vi "Calculate_Angles_Locally_Optimum-1.vi"(4 "Statuses":i16[](array[numeric]), 5 "[IN] Index of subtrack":i32, 6 "[IN] Reverse Displ or Not":bool[](array[boolean]), 7 "[IN] Array with Angles \nBetween Displacement":dbl[](array[numeric]), 8 "[IN] Index of Cur\nrent Displacement":i32, 9 "[IN] Track with \nCurrent Point":dbl[](array[numeric]), 10 "[IN] Index of Previ\nous Displacement":i32, 11 "[IN] Track with \nPrevious Point":dbl[](array[numeric])) -> (1 "[OUT] Reverse displacement or not":bool[](array[boolean]), 2 "[OUT] Angles betwe\nen two displacements":dbl[](array[numeric]))   [LabVIEW 2013]
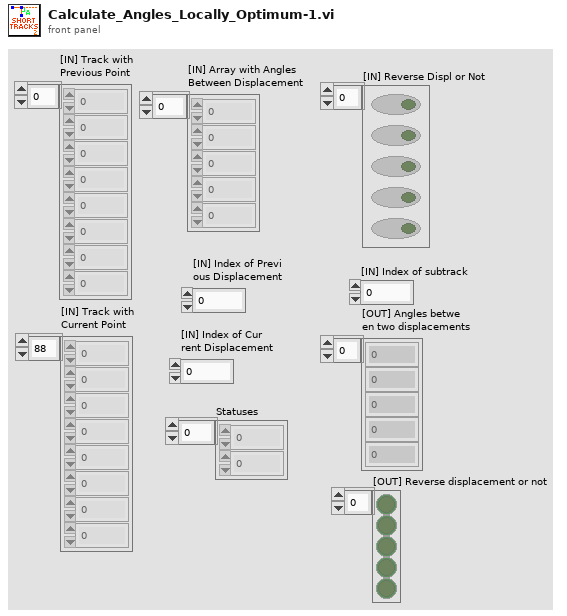
[diagram p1: front panel]
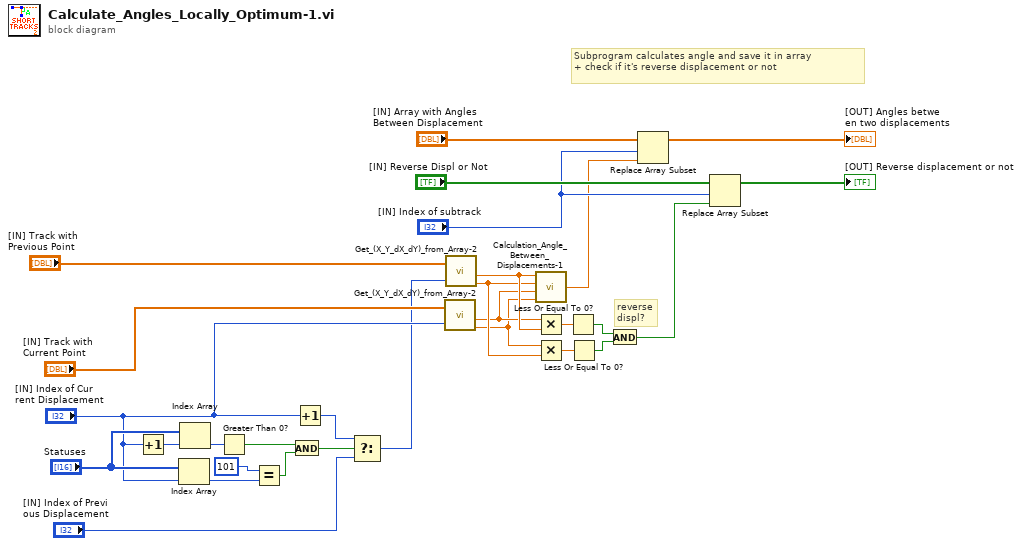
[diagram p0: block diagram]
diagram:
  # "Subprogram calculates angle and save it in array \n+ check if it's reverse displacement or not"
  # "reverse \ndispl?"
  n1 = Increment(x="[IN] Index of Cur\nrent Displacement") -> (x+1=w14:i32)
  n2 = Index Array(array="Statuses", index="[IN] Index of Cur\nrent Displacement") -> (element=w17:i16)
  n3 = Index Array(array="Statuses", index=w14) -> (element=w13:i16)
  n4 = Greater Than 0?(x=w13) -> (x > 0?=w12:bool)
  n5 = Equal?(x=i16 101, y=w17) -> (x = y?=w11:bool)
  n6 = And(x=w12, y=w11) -> (x .and. y?=w10:bool)
  n7 = Increment(x="[IN] Index of Cur\nrent Displacement") -> (x+1=w8:i32)
  n8 = Select(t=w8, s=w10, f="[IN] Index of Previ\nous Displacement") -> (s? t:f=w6:i32)
  n9 = call "Get_(X_Y_dX_dY)_from_Array-2.vi"("(X,Y,dX,dY)"="[IN] Track with \nCurrent Point", "Index of Displacement"="[IN] Index of Cur\nrent Displacement") -> ("dX"=w3:dbl, "dY"=w2:dbl)  [unwired: 2 out]
  n10 = call "Get_(X_Y_dX_dY)_from_Array-2.vi"("(X,Y,dX,dY)"="[IN] Track with \nPrevious Point", "Index of Displacement"=w6) -> ("dX"=w5:dbl, "dY"=w4:dbl)  [unwired: 2 out]
  n11 = call "Calculation_Angle_Between_Displacements-1.vi"("dY 2"=w2, "dX 2"=w3, "dY 1"=w4, "dX 1"=w5) -> ("angle in degrees"=w1:dbl)
  n12 = Multiply(x=w3, y=w5) -> (x*y=w28:dbl)
  n13 = Multiply(x=w2, y=w4) -> (x*y=w27:dbl)
  n14 = Less Or Equal To 0?(x=w28) -> (x <= 0?=w25:bool)
  n15 = Less Or Equal To 0?(x=w27) -> (x <= 0?=w26:bool)
  n16 = And(x=w25, y=w26) -> (x .and. y?=w21:bool)
  n17 = Replace Array Subset(array="[IN] Array with Angles \nBetween Displacement", new element=w1, index="[IN] Index of subtrack") -> (→"[OUT] Angles betwe\nen two displacements":dbl[])
  n18 = Replace Array Subset(array="[IN] Reverse Displ or Not", new element=w21, index="[IN] Index of subtrack") -> (→"[OUT] Reverse displacement or not":bool[])
